vi "AOI Stats.vi"(6 "Params In":T1(array[cluster]) {"Value" format="%.2f"}, 8 "error in":errorcluster, 9 "AOI (l, t, r, b)":u16[](array[numeric]), 10 "Image Type":u32, 11 "Image In":T2) -> (0 "error out":errorcluster, 1 "integral":i32, 3 "Image Out":T2, 4 "Params out":T1(array[cluster]) {"Value" format="%.2f"})   [LabVIEW 2011]
uses:
  <vilib>/vision/Image Controls.llb/IMAQ Image.ctl
  <vilib>/vision/NI_Vision_Development_Module.lvlib
panel:
  out "threshold":i16
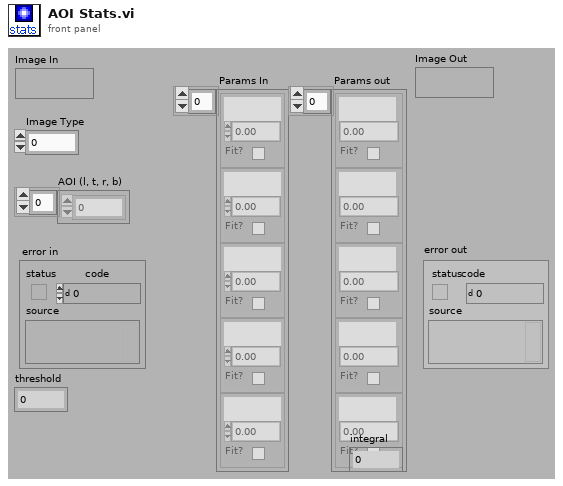
[diagram p1: front panel]
types:
  T1 = cluster{"Name":string, "Value":dbl, "Fit?":bool}[]
  T2 = typedef "IMAQ Image.ctl" = refnum<image>
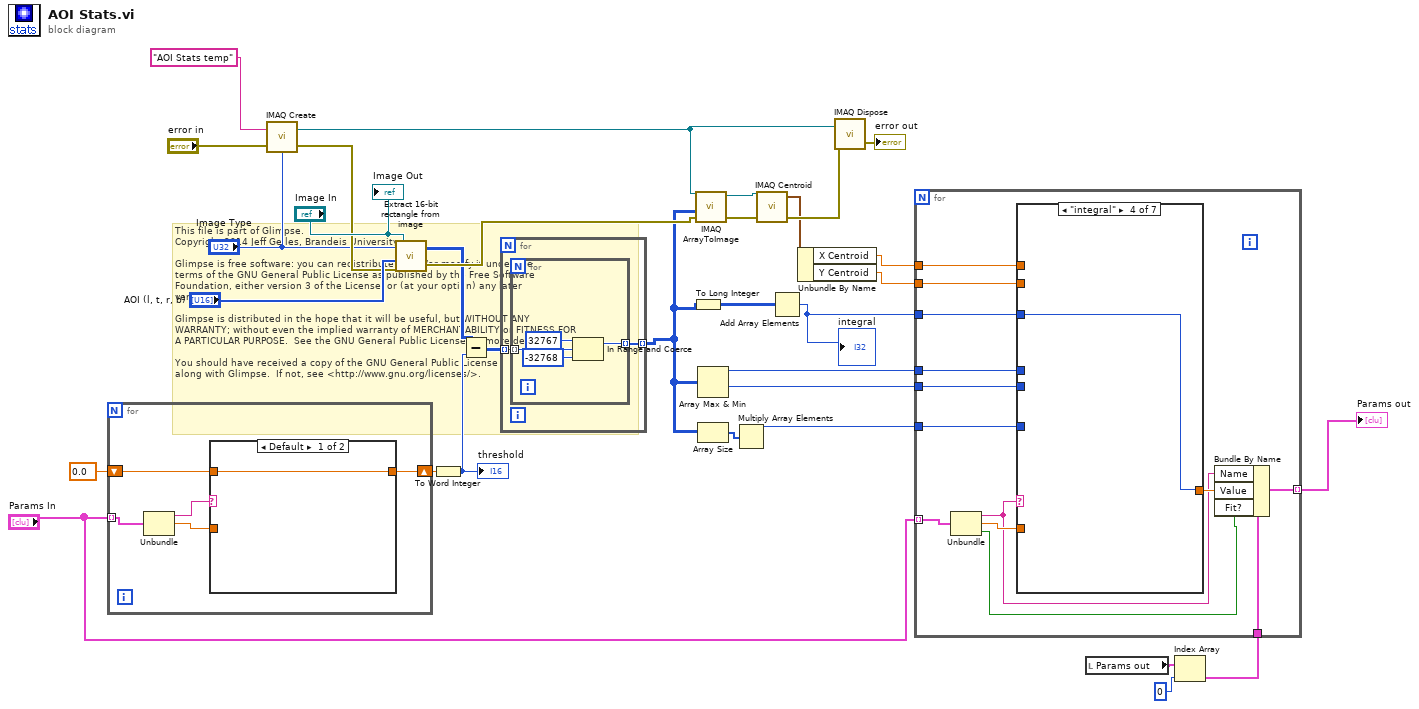
[diagram p0: block diagram]
diagram:
  # "This file is part of Glimpse. \nCopyright 2014 Jeff Gelles, Brandeis University.    \n\nGlimpse is free software: you can redistribute it and/or modify it under the \nterms of the GNU General Public License as published by the Free Software \nFoundation, either version 3 of the License, or (at your option) any later \nversion.\n\nGlimpse is distributed in the hope that it will be useful, but WITHOUT ANY \nWARRANTY; without even the implied warranty of MERCHANTABILITY or FITNESS FOR \nA PARTICULAR PURPOSE.  See the GNU General Public License for more details.\n\nYou should have received a copy of the GNU General Public License\nalong with Glimpse.  If not, see <http://www.gnu.org/licenses/>."
  n1 = for {
    tunnel: "Params In" -> [w37] mode=indexing
    shift-right: [w34] -> w29
    shift-left: 0.0 ("Value") -> [w33]
    n2 = Unbundle(w37) -> ("Name"=w36:string, "Value"=w35:dbl)  [unwired: 1 out]
    n3 = case shown="Default" w36 {
      tunnel: w35 -> [_ w39]
      tunnel: [w38 w39] -> w34
      tunnel: w33 -> [w38 _]
      frame Default {
      }
      frame "threshold" {
      }
    }
  }
  n4 = call "IMAQ Create"("Image Name"="AOI Stats temp", "Image Type"="Image Type", "error in (no error)"="error in") -> ("New Image"=w17:T2, "error out"=w25:errorcluster)  [unwired: 1 in, 1 out]
  n5 = call "Extract 16-bit rectangle from image.vi"("error in"=w25, "AOI (t, l, b, r)"="AOI (l, t, r, b)", "Image pixel depth"="Image Type", "Image in"="Image In") -> ("error out"=w22:errorcluster, "Image Pixels (I16)"=w19:i16[][])
  n6 = To Word Integer(number=w29) -> (16bit integer=w28:i16)
  "threshold" <- w28
  n7 = Subtract(x=w19, y=w28) -> (x-y=w2:i16[][])
  n8 = for {
    tunnel: w2 -> [w41] mode=indexing
    tunnel: [w40] -> w1 mode=indexing
    n9 = for {
      tunnel: w41 -> [w45] mode=indexing
      tunnel: [w44] -> w40 mode=indexing
      n10 = In Range and Coerce(upper limit=i16 32767, x=w45, lower limit=i16 -32768) -> (coerced(x)=w44:i16)  [unwired: 1 out]
    }
  }
  n11 = To Long Integer(number=w1) -> (32bit integer=w3:i32[][])
  n12 = call "IMAQ ArrayToImage"("error in (no error)"=w22, "Image Pixels (I16)"=w1, "Image"=w17) -> ("error out"=w20:errorcluster, "Image Out"=w21:T2)  [unwired: 3 in, 4 out]
  n13 = Array Max & Min(array=w1) -> (max value=w11:i16, min value=w10:i16)  [unwired: 2 out]
  n14 = Array Size(array=w1) -> (size(s)=w8:i32[])
  n15 = Multiply Array Elements(1:w8) -> (0:w7:i32)
  n16 = call "IMAQ Centroid"("error in (no error)"=w20, "Image"=w21) -> ("error out"=w18:errorcluster, "Centroid"=w15:cluster{"X Centroid":sgl, "Y Centroid":sgl})  [unwired: 1 in, 1 out]
  n17 = Add Array Elements(numeric array=w3) -> (sum=w12:i32)
  "integral" <- w12
  n18 = Unbundle By Name(w15) -> ("X Centroid"=w14:sgl, "Y Centroid"=w13:sgl)
  n19 = call "IMAQ Dispose"("Image"=w17, "error in (no error)"=w18) -> ("error out"=→"error out":errorcluster)  [unwired: 1 in, 3 out]
  n20 = local read "Params out"() -> (w6:T1)
  n21 = Index Array(array=w6, index=0) -> (element=w4:cluster{"Name":string, "Value":dbl, "Fit?":bool})
  n22 = for {
    tunnel: "Params In" -> [w49] mode=indexing
    tunnel: [w56] -> w16 mode=indexing
    tunnel: w14 -> [w55]
    tunnel: w13 -> [w54]
    tunnel: w12 -> [w53]
    tunnel: w11 -> [w52]
    tunnel: w10 -> [w51]
    tunnel: w7 -> [w50]
    tunnel: w4 -> [w48]
    n23 = Unbundle(w49) -> ("Name"=w47:string, "Value"=w58:dbl, "Fit?"=w46:bool)
    n24 = case shown="\"integral\"" w47 {
      tunnel: w58 -> [w59 _ _ _ _ _ _]
      tunnel: [w59 w60 w61 w62 w63 w64 w65] -> w57
      tunnel: w55 -> [_ w60 _ _ _ _ _]
      tunnel: w54 -> [_ _ w61 _ _ _ _]
      tunnel: w53 -> [_ _ _ w62 _ _ _]
      tunnel: w52 -> [_ _ _ _ w63 _ _]
      tunnel: w51 -> [_ _ _ _ _ w64 _]
      tunnel: w50 -> [_ _ _ _ _ _ w65]
      frame Default {
      }
      frame "xc" {
      }
      frame "yc" {
      }
      frame "integral" {
      }
      frame "max" {
      }
      frame "min" {
      }
      frame "npix" {
      }
    }
    n25 = Bundle By Name(cluster=w48, "Name"=w47, "Value"=w57, "Fit?"=w46) -> (w56:cluster{"Name":string, "Value":dbl, "Fit?":bool})
  }
  "Params out" <- w16
  "Image Out" <- "Image In"
